vi "RichToFlatnixnet_grpc_DbGetDBCAttributeResponse.vi"(5 "OutputClusterType":T1, 11 "InputCluster":T2) -> (3 "OutputCluster":T1)   [LabVIEW 2025, in "grpc-xnet_client.lvlib"]
uses:
  nixnet_grpc_DbGetDBCAttributeResponse.ctl
  nixnet_grpc_DbGetDBCAttributeResponse_Flat.ctl
  grpc-xnet_client.lvlib
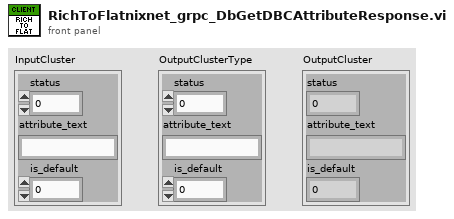
[diagram p1: front panel]
types:
  T1 = typedef "grpc-xnet_client.lvlib/nixnet_grpc_DbGetDBCAttributeResponse_Flat.ctl" = cluster{"status":i32, "attribute_text":string, "is_default":u32}
  T2 = typedef "grpc-xnet_client.lvlib/nixnet_grpc_DbGetDBCAttributeResponse.ctl" = cluster{"status":i32, "attribute_text":string, "is_default":u32}
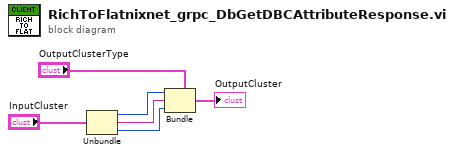
[diagram p0: block diagram]
diagram:
  n1 = Unbundle "Unbundle"("InputCluster") -> ("status"=w3:i32, "attribute_text"=w2:string, "is_default"=w1:u32)
  n2 = Bundle "Bundle"(cluster="OutputClusterType", "status"=w3, "attribute_text"=w2, "is_default"=w1) -> (→"OutputCluster":T1)
